vi "WSVCAP SHL Host TL Tester.vi"(0 "FPGA":T4) -> ()   [LabVIEW 2017]
uses:
  WSVCAP Shell Host Low Level/Host SRL/Type Defs/Cycle Pair Cluster.ctl
  Type Defs/WSVCAP SHL DUT Number Enum.ctl
  <vilib>/userdefined/High Color/nirio_resource_hc.ctl
  Type Defs/WSVCAP SHL FPGA Enum.ctl
  WSVCAP Shell Host Low Level/Host SRL/Type Defs/Cycle Instruction Cluster.ctl
  WSVCAP Shell Host Low Level/Host SRL/Type Defs/Cycle Scheme Enum.ctl
  Type Defs/Cap and DAC Table Manager Operation Enum.ctl
  Type Defs/WSVCAP SHL I2C DUT Mask Mode Enum.ctl
  WSVCAP Shell FPGA Low Level/FPGA-SRL/Debug Global.vi
  Type Defs/WSVCAP SHL Tester System Cluster.ctl
  WSVCAP Shell Host Low Level/Host SRL/Host SRL.lvlib
  WSVCAP Shell FPGA Low Level/FPGA-SRL/FPGA-SRL.lvlib
panel:
  in  "Cycle Scheme":T1
  in  "Cycle Pairs":T2[](array[typedef])=[{"G1 Ch (0-5)"=1, "G2 Ch (0-5)"=0, "En"=TRUE}, {"G1 Ch (0-5)"=3, "G2 Ch (0-5)"=2, "En"=TRUE}, {"G1 Ch (0-5)"=4, "G2 Ch (0-5)"=5, "En"=TRUE}] {"G2 Ch (0-5)" max=5 step=1 format="Ch %.0f"; "G1 Ch (0-5)" max=5 step=1 format="Ch %.0f"}
  in  "Vout 2 (V)":dbl=44.0 caption="Vout 2" format="%.3f V"
  in  "Device Ch (0-23)":u32
  in  "Data Out (14-bit)":u16 format="0x%04x"
  in  "Delay 2 (s)":dbl=5e-05 caption="Delay 2" format="%#_4ps"
  in  "Delay 1 (s)":dbl=5e-05 caption="Delay 1" format="%#_4ps"
  in  "Vout 1 (V)":dbl=44.0 caption="Vout 1" format="%.3f V"
  out "Cycle Count":u64=2 min=1 max=4 step=1
  out "Cycle Instructions":T3[](array[typedef]) {"Post CMD Delay (s)" format="%#_4ps"; "DAC Vout (V)" format="%.3f V"; "Dev Ch Idx (0-5)" max=5 step=1 format="Ch %d"}
  in  "Device Idx (0-5)":u32
  out "Dev Ch Idx (0-31)":u32 max=5 step=1 format="Dev Ch Idx: %d"
  out "Dev Idx (0-5)":u32 max=5 step=1 format="Dev Idx: %d"
  in  "DAC Out Vref (V)":dbl format="%.3f V"
  out "CMD [Hex]":u32 max=5 step=1 format="0x%05x"
  out "CMD [Bin]":u32 max=5 step=1 format="0b%019b"
  in  "Write DAC Voltage":bool
  in  "DUT Ch Idx (0-5)":u32 caption="DUT Ch Idx" max=5 step=1
  in  "DAC Vout (V)":dbl caption="Vout" format="%.3f V"
  in  "Cap DAC":u8=144 caption="B Data In" format="0x%02x"
  in  "Set Cap DAC":bool
  in  "Write Raw SRL":bool
  in  "Write Data DUT":string caption="Write Data Out"
  in  "Stop SRL Cycle":bool
  in  "Start SRL Cycle":bool
  in  "Monitor":bool
  out "AD7747 Values":string[][](table)
  in  "Mode":enum32{"All", "Single"}(radio)
  out "Activity Log":string
  out "Simulate FPGA":bool
  out "Online":bool
  out "FPGA Resource":T5
  out "Status":string
  out "Busy":bool
  in  "I2C Bytes to Read":u8=1 caption="Bytes" min=1 max=4 step=1
  in  "Exit":bool
  out "Read Data I2C":u8[](array[numeric]) caption="Data In" format="0x%02x"
  in  "Read Reg I2C":u8 caption="Register" format="0x%02x"
  in  "Read I2C":bool
  in  "DUT":T6
  in  "Write Data I2C":u8 caption="Data Out" format="0x%02x"
  in  "Write Reg I2C":u8=144 caption="Register" format="0x%02x"
  in  "I2C Init":bool
  in  "Init Data":u8[](array[numeric])=[164, 160, 14, 33] caption="Data Out" format="0x%02x"
  in  "Init Reg":u8[](array[numeric])=[191, 7, 9, 10] caption="Register" format="0x%02x"
  in  "Write I2C":bool
  in  "I2C Slave Address":u8=144 caption="Slave Address" format="0x%02x"
  in  "SRL Clock Rate (Hz)":dbl=1000000.0 caption="Clock Rate" format="%.1p Hz"
  in  "I2C Clock Rate (Hz)":dbl=100000.0 caption="Clock Rate" format="%.0p Hz"
  in  "Error":errorcluster
  # "WS1021 MEMS Only Tester"
  # "AD7747 (I2C)"
  # "C"
  # "DAC Control (SRL)"
  # "Vout Cycling (SRL)"
  # "Group 1"
  # "Group 2"
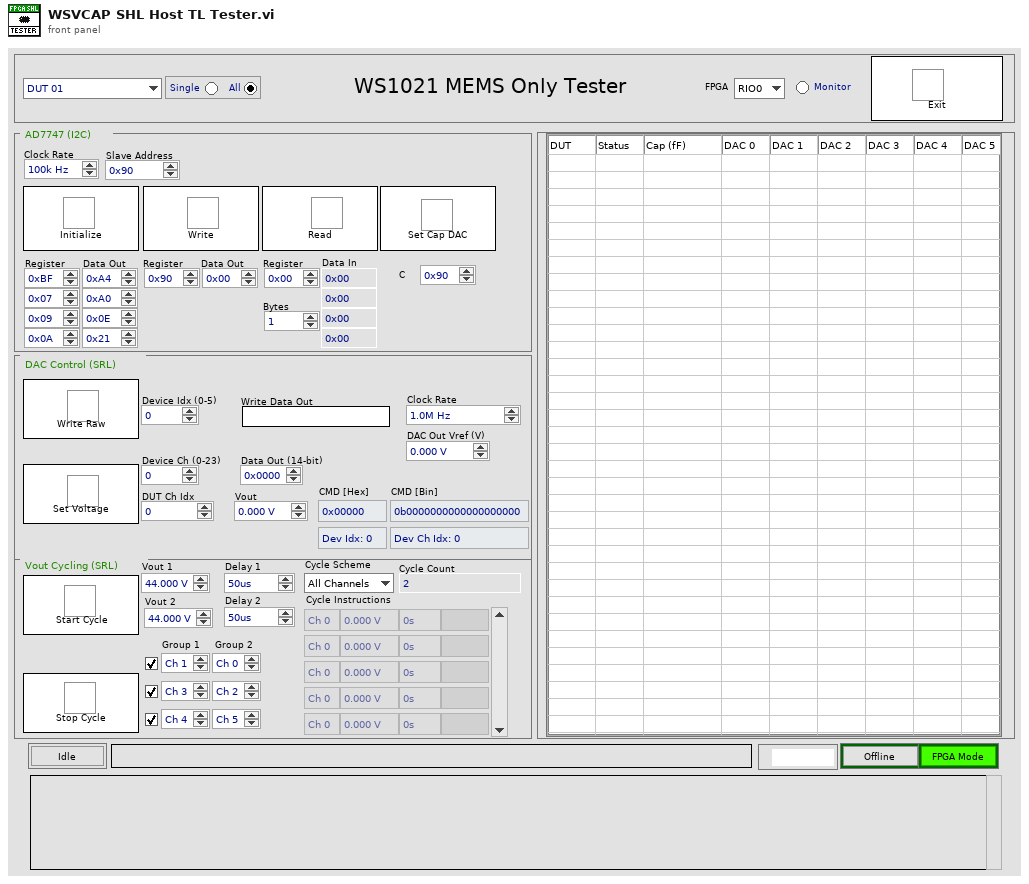
[diagram p1: front panel]
types:
  T1 = typedef "Cycle Scheme Enum.ctl" = enum16{"All Channels", "By Group"}
  T2 = typedef "Host SRL.lvlib/Cycle Pair Cluster.ctl" = cluster{"G1 Ch (0-5)":u32, "G2 Ch (0-5)":u32, "En":bool}
  T3 = typedef "Host SRL.lvlib/Cycle Instruction Cluster.ctl" = cluster{"Dev Ch Idx (0-5)":u32, "DAC Vout (V)":dbl, "Post CMD Delay (s)":dbl, "Raw CMD":string}
  T4 = typedef "WSVCAP SHL FPGA Enum.ctl" = enum16{"RIO0", "RIO1"}
  T5 = typedef "nirio_resource_hc.ctl" = tag
  T6 = typedef "WSVCAP SHL DUT Number Enum.ctl" = enum16{"DUT 01", "DUT 02", "DUT 03", "DUT 04", "DUT 05", "DUT 06", "DUT 07", "DUT 08", "DUT 09", "DUT 10", "DUT 11", "DUT 12", "DUT 13", "DUT 14", "DUT 15", "DUT 16", "DUT 17", "DUT 18", "DUT 19", "DUT 20", "DUT 21", "DUT 22", "DUT 23", "DUT 24"}
  T7 = typedef "Cap and DAC Table Manager Operation Enum.ctl" = enum16{"Initialize", "Add Single DAC", "Add All DAC", "Add All DUT Single DAC", "Add All Cap", "Get Status"}
  T8 = typedef "WSVCAP SHL Core System Cluster.ctl" = cluster{"Settings":T9, "FPGA Resource":tag, "Online":bool, "I2C Wait Ticks":u32, "SRL Wait Ticks":u32, "FPGA VI Reference (FPGA Mode)":T10, "FPGA VI Reference (Sim Mode)":refnum<vi>}
  T9 = typedef "WSVCAP SHL I2C Settings Cluster.ctl" = cluster{"I2C Slave Address":u8, "I2C Clock Rate (Hz)":dbl, "SRL Clock Rate (Hz)":dbl, "Simulate FPGA":bool, "C1 Cap DAC Default":u8, "C2 Cap DAC Default":u8, "C3 Cap DAC Default":u8, "C4 Cap DAC Default":u8, "DAC Out Vref (V)":dbl}
  T10 = typedef "WSVCAP SHL FPGA Ref.ctl" = refnum<k20>
  T11 = enum8{"Enabled", "Disabled", "Disabled and Grayed Out"}
  T12 = typedef "WSVCAP SHL I2C DUT Mask Mode Enum.ctl" = enum16{"Custom", "All"}
  T13 = typedef "WSVCAP SHL Tester System Cluster.ctl" = cluster{"I2C Monitor":bool, "SRL Cyle":bool, "DAC Vout (V)":dbl, "DUT Ch Idx (0-5)":u32, "Cycle Instructions":T3[], "Vout 1 (V)":dbl, "Delay 1 (s)":dbl, "Number of pairs":i32, "Delay 2 (s)":dbl, "Data Out (14-bit)":u16, "DUT":T6, "Vout 2 (V)":dbl, "Cycle Scheme":T1}
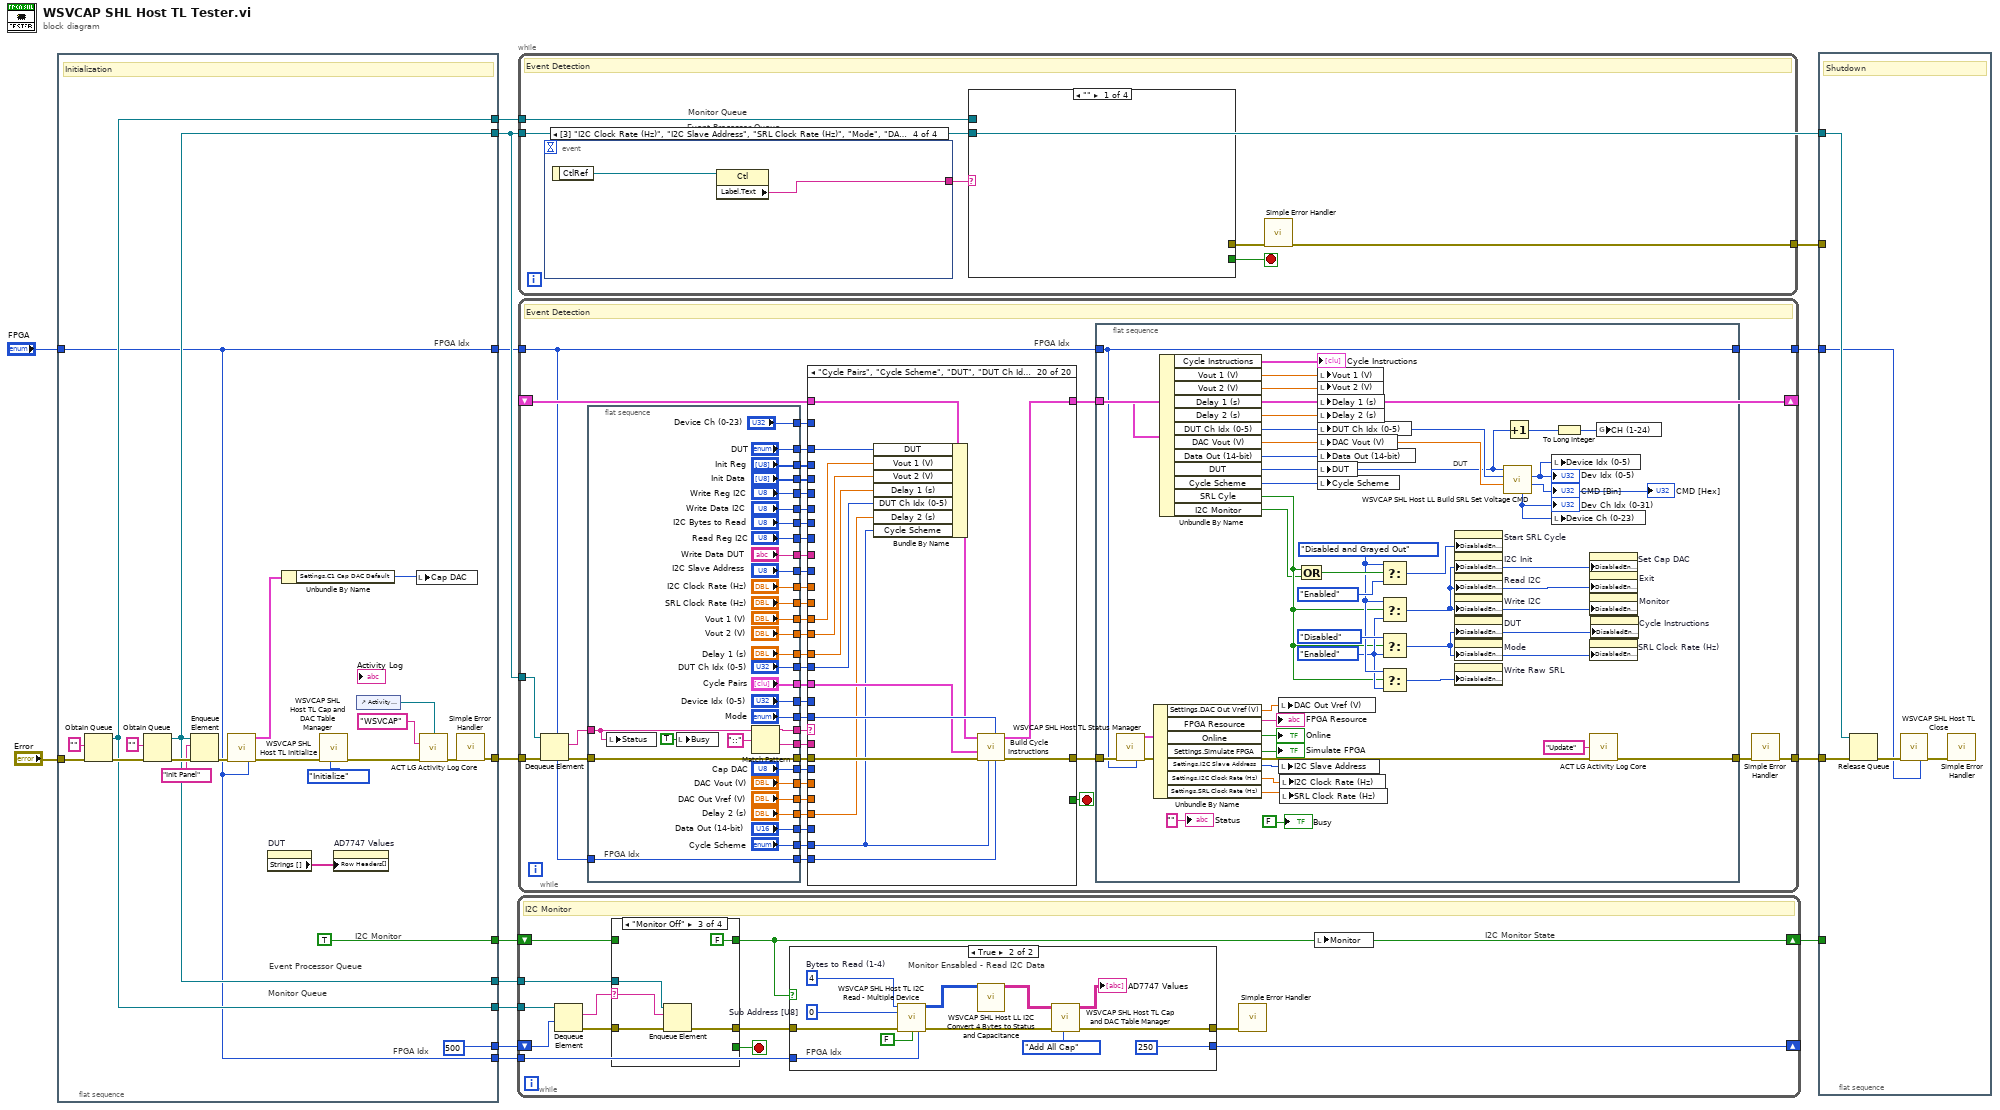
[diagram p0: block diagram]
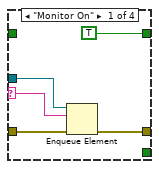
[diagram p2: hidden frame]
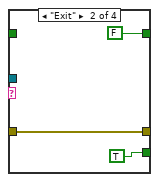
[diagram p3: hidden frame]
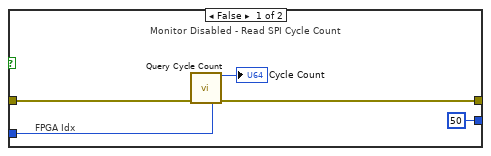
[diagram p5: hidden frame]
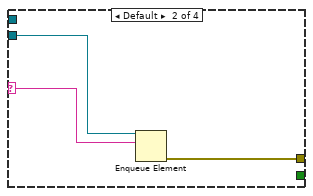
[diagram p6: hidden frame]
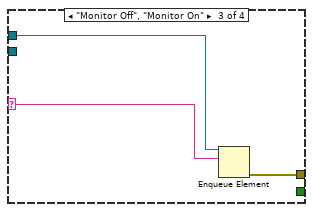
[diagram p7: hidden frame]
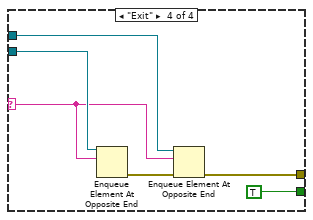
[diagram p8: hidden frame]
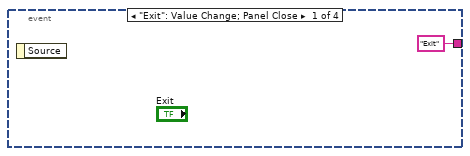
[diagram p9: hidden frame]
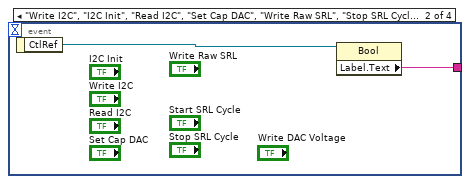
[diagram p10: hidden frame]
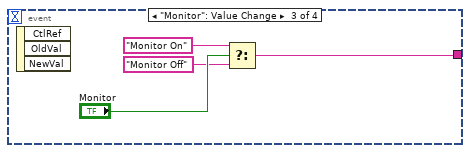
[diagram p11: hidden frame]
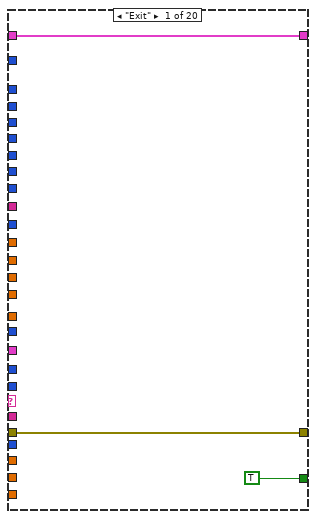
[diagram p12: hidden frame]
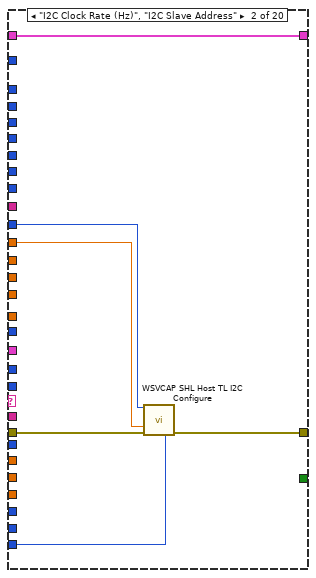
[diagram p13: hidden frame]
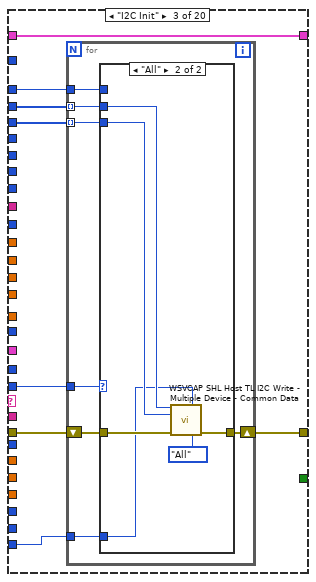
[diagram p14: hidden frame]
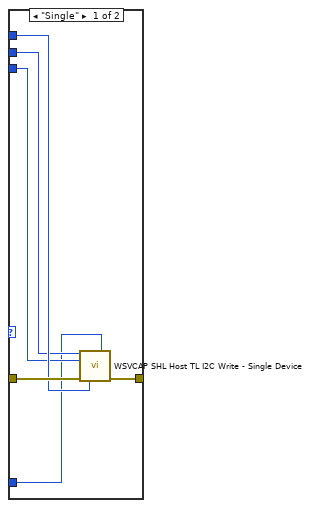
[diagram p15: hidden frame]
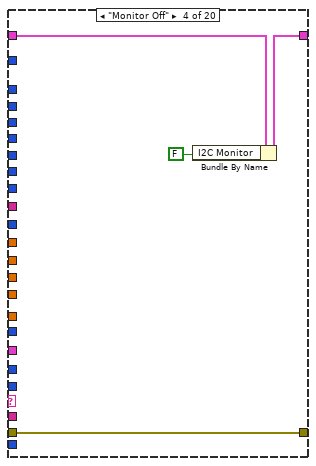
[diagram p16: hidden frame]
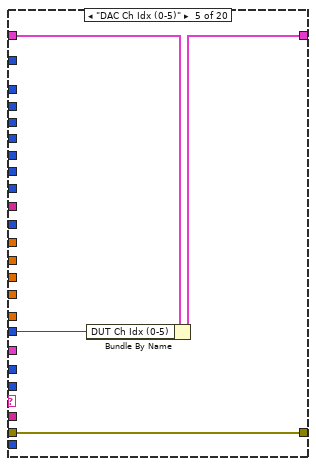
[diagram p17: hidden frame]
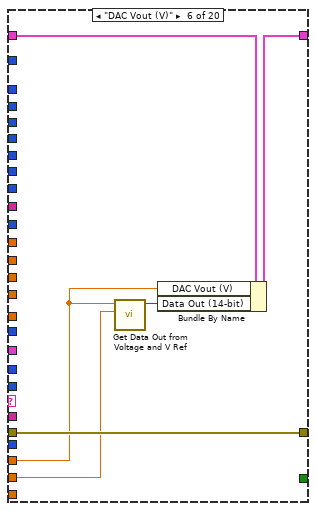
[diagram p18: hidden frame]
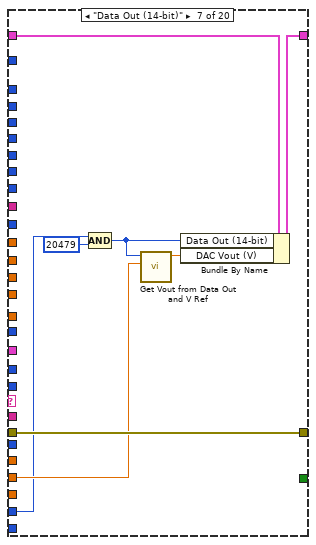
[diagram p19: hidden frame]
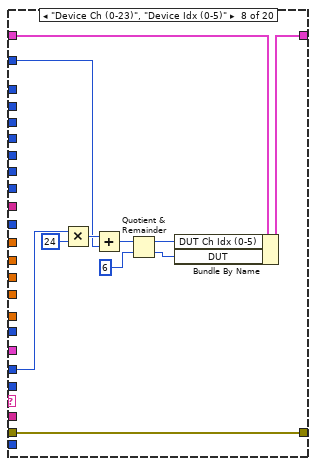
[diagram p20: hidden frame]
diagram:
  n1 = flat-sequence "Initialize" {
    tunnel: "Error" -> [w28]
    tunnel: [w26] -> w14
    tunnel: [TRUE ("Monitor")] -> w7
    tunnel: [w33] -> w11
    tunnel: [w25] -> w10
    tunnel: [w26] -> w9
    tunnel: [w25] -> w8
    tunnel: [500 ("Wait Time (500ms)")] -> w6
    tunnel: "FPGA" -> [w19]
    tunnel: [w19] -> w4
    tunnel: [w19] -> w2
    frame #0 {
      # "FPGA Idx"
      # "FPGA Idx"
      # "I2C Monitor"
      # "Monitor Queue"
      # "Event Processor Queue"
      # "Initialization"
      n2 = Obtain Queue(element data type="" ("name (unnamed)"), error in (no error)=w28) -> (queue out=w25:refnum<queue>, error out=w27:errorcluster)  [unwired: 3 in, 1 out]
      n3 = Obtain Queue(element data type="" ("name (unnamed)"), error in (no error)=w27) -> (queue out=w26:refnum<queue>, error out=w36:errorcluster)  [unwired: 3 in, 1 out]
      n4 = Enqueue Element(queue=w26, element="Init Panel" ("name (unnamed)"), error in (no error)=w36) -> (error out=w23:errorcluster)  [unwired: 1 in, 2 out]
      n5 = call "WSVCAP SHL Host TL Initialize.vi"("error in"=w23, "FPGA"=w19) -> ("System"=w22:T8, "error out"=w17:errorcluster)  [unwired: 12 in]
      n6 = property on="DUT" class="Enum (strict)"() -> ("Strings []"=w24:string[])  [unwired: 2 in, 2 out]
      n7 = Unbundle By Name(w22) -> ("Settings.C1 Cap DAC Default"=w21:u8)
      n8 = call "WSVCAP SHL Host TL Cap and DAC Table Manager.vi"("Operation"=Cap_and_DAC_Table_Manager_Operation_Enum."Initialize", "Error In"=w17) -> ("Error Out"=w16:errorcluster)  [unwired: 8 in, 1 out]
      n9 = property on="AD7747 Values" class="Tbl (strict)"("Row Headers[]"=w24) -> ()  [unwired: 2 in, 2 out]
      n10 = control-ref of="Activity Log"() -> (w32:refnum<vi>)
      n11 = local write "Cap DAC"(w21) -> ()
      n12 = call "ACT LG Activity Log Core.vi"("Display Ref"=w32, "Source"="WSVCAP", "Error In (no error)"=w16) -> ("Error Out"=w34:errorcluster)  [unwired: 11 in, 1 out]
      n13 = call <vilib>:"Simple Error Handler.vi"("error in (no error)"=w34) -> ("error out"=w33:errorcluster)  [unwired: 4 in, 4 out]
    }
  }
  n14 = while "Monitor" {
    shift-right: [w41] -> w1
    shift-left: w7 -> [w47]
    tunnel: w10 -> [w45]
    tunnel: w9 -> [w44]
    shift-right: [w40] -> _
    shift-left: w6 -> [w39]
    tunnel: w2 -> [w38]
    stop <- w42 stop-if-true
    # "I2C Monitor State"
    # "I2C Monitor"
    n15 = Dequeue Element(queue=w45, timeout in ms (-1)=w39) -> (element=w48:string, error out=w46:errorcluster)  [unwired: 1 in, 2 out]
    n16 = case shown="\"Monitor Off\"" w48 {
      selector: w48 -> [w51 _ w59 _]
      tunnel: [TRUE FALSE FALSE w64] -> w41
      tunnel: w47 -> [_ _ _ w64]
      tunnel: w46 -> [w53 w56 w61 w63]
      tunnel: [w52 w56 w60 w63] -> w43
      tunnel: w44 -> [w50 _ w58 _]
      tunnel: [_ TRUE _ _] -> w42
      frame "Monitor On" {
        n17 = Enqueue Element(queue=w50, element=w51, error in (no error)=w53) -> (error out=w52:errorcluster)  [unwired: 1 in, 2 out]
      }
      frame "Exit" {
      }
      frame "Monitor Off" {
        n18 = Enqueue Element(queue=w58, element=w59, error in (no error)=w61) -> (error out=w60:errorcluster)  [unwired: 1 in, 2 out]
      }
      frame Default {
      }
    }
    n19 = case shown="True" w41 {
      tunnel: [w67 w71] -> w49
      tunnel: w43 -> [w68 w78]
      tunnel: [50 ("Wait Time (500ms)") 250 ("Wait Time (500ms)")] -> w40
      tunnel: w38 -> [w65 w75]
      frame False {
        # "FPGA Idx"
        # "Monitor Disabled - Read SPI Cycle Count"
        n20 = call "Query Cycle Count.vi"("error in"=w68, "FPGA"=w65) -> ("Cycle Count"=→"Cycle Count":u64, "error out"=w67:errorcluster)  [unwired: 12 in]
      }
      frame True {
        w80 = u8 4  # Bytes to Read (1-4)
        w81 = u8 0  # Sub Address [U8]
        # "FPGA Idx"
        # "Monitor Ensabled - Read I2C Data"
        n21 = call "WSVCAP SHL Host TL I2C Read - Multiple Device.vi"("Bytes to Read (1-4)"=w80, "Sub Address [U8]"=w81, "error in"=w78, "Log (T)"=FALSE, "FPGA"=w75) -> ("C:1-24 Read Data [U8]"=w79:u8[][], "error out"=w72:errorcluster)  [unwired: 9 in]
        n22 = call "WSVCAP SHL Host LL I2C Convert 4 Bytes to Status and Capacitance.vi"("C:1-24 Read Data [U8]"=w79) -> ("AD7747 Values"=w74:string[][])  [unwired: 14 in]
        n23 = call "WSVCAP SHL Host TL Cap and DAC Table Manager.vi"("Operation"=Cap_and_DAC_Table_Manager_Operation_Enum."Add All Cap", "Error In"=w72, "Data In"=w74) -> ("Error Out"=w71:errorcluster, "Table Out"=→"AD7747 Values":string[][])  [unwired: 7 in]
      }
    }
    n24 = call <vilib>:"Simple Error Handler.vi"("error in (no error)"=w49) -> ()  [unwired: 4 in, 5 out]
    n25 = local write "Monitor"(w41) -> ()
  }
  n26 = while "User Interface Event Detector" {
    tunnel: w14 -> [w86]
    tunnel: [w83] -> w12
    tunnel: w8 -> [w82]
    stop <- w84 stop-if-true
    # "Monitor Queue"
    # "Event Processor Queue"
    # "Event Detection"
    n27 = event shown="[3] \"I2C Clock Rate (Hz)\", \"I2C Slave Address\", \"SRL Clock Rate (Hz)\", \"Mode\", \"DAC Out Vref (V)\", \"DUT Ch Idx (0-5)\", \"DAC Vout (V)\", \"DUT\", \"Vout 1 (V)\", \"Delay 1 (s)\", \"Cycle Pairs\", \"Data Out (14-bit)\", \"Device Ch (0-23)\", \"Delay 2 (s)\", \"Vout 2 (V)\", \"Cycle Scheme\": Value Change" {
      selector: _ -> [_ _ _ _]
      dyn-events: _ -> [_ _ _ _]
      timeout: _ -> [_ _ _ _]
      tunnel: ["Exit" ("Label.Text") w102 w103 w107] -> w87
      event "Exit": Value Change; Panel Close {
        n28 = event-data() -> ()  [unwired: 1 in, 1 out]
      }
      event "Write I2C", "I2C Init", "Read I2C", "Set Cap DAC", "Write Raw SRL", "Stop SRL Cycle", "Start SRL Cycle", "Write DAC Voltage": Value Change {
        n29 = event-data() -> ("CtlRef"=w101:refnum<vi>)  [unwired: 1 in]
        n30 = property class="Bool"(reference=w101) -> ("Label.Text"=w102:string)  [unwired: 1 in, 2 out]
      }
      event "Monitor": Value Change {
        n31 = event-data() -> ()  [unwired: 1 in, 3 out]
        n32 = Select(t="Monitor On" ("Label.Text"), s="Monitor", f="Monitor Off" ("Label.Text")) -> (s? t:f=w103:string)
      }
      event "I2C Clock Rate (Hz)", "I2C Slave Address", "SRL Clock Rate (Hz)", "Mode", "DAC Out Vref (V)", "DUT Ch Idx (0-5)", "DAC Vout (V)", "Vout 1 (V)", "Delay 1 (s)", "Cycle Pairs", "Data Out (14-bit)", "Device Ch (0-23)", "Delay 2 (s)", "Vout 2 (V)": Value Change {
        n33 = event-data() -> ("CtlRef"=w108:refnum<vi>)  [unwired: 1 in]
        n34 = property class="Ctl"(reference=w108) -> ("Label.Text"=w107:string)  [unwired: 1 in, 2 out]
      }
    }
    n35 = case shown="\"\"" w87 {
      selector: w87 -> [_ w90 w93 w94]
      tunnel: w86 -> [_ w89 _ w99]
      tunnel: [_ w88 w92 w96] -> w85
      tunnel: [_ _ _ TRUE] -> w84
      tunnel: w82 -> [_ _ w91 w95]
      frame "" {
      }
      frame Default {
        n36 = Enqueue Element(queue=w89, element=w90) -> (error out=w88:errorcluster)  [unwired: 2 in, 2 out]
      }
      frame "Monitor Off", "Monitor On" {
        n37 = Enqueue Element(queue=w91, element=w93) -> (error out=w92:errorcluster)  [unwired: 2 in, 2 out]
      }
      frame "Exit" {
        n38 = Enqueue Element At Opposite End(queue=w99, element=w94) -> (error out=w97:errorcluster)  [unwired: 2 in, 2 out]
        n39 = Enqueue Element At Opposite End(queue=w95, element=w94, error in (no error)=w97) -> (error out=w96:errorcluster)  [unwired: 1 in, 2 out]
      }
    }
    n40 = call <vilib>:"Simple Error Handler.vi"("error in (no error)"=w85) -> ("error out"=w83:errorcluster)  [unwired: 4 in, 4 out]
  }
  n41 = while "Event Processer" {
    tunnel: w14 -> [w149]
    tunnel: [w147] -> w13
    tunnel: w11 -> [w130]
    shift-right: [w128] -> _
    shift-left: _ -> [w129]
    tunnel: w4 -> [w123]
    tunnel: [w109] -> w3
    stop <- w148 stop-if-true
    # "FPGA Idx"
    # "Event Detection"
    n42 = Dequeue Element(queue=w149, error in (no error)=w130) -> (element=w145:string, error out=w143:errorcluster)  [unwired: 1 in, 2 out]
    n43 = flat-sequence {
      tunnel: ["I2C Clock Rate (Hz)"] -> w146
      tunnel: [w208] -> w144
      tunnel: w145 -> [w209]
      tunnel: [w222] -> w142
      tunnel: w143 -> [w222]
      tunnel: ["I2C Bytes to Read"] -> w141
      tunnel: ["I2C Slave Address"] -> w140
      tunnel: ["SRL Clock Rate (Hz)"] -> w139
      tunnel: ["DUT"] -> w122
      tunnel: ["Init Data"] -> w136
      tunnel: ["Init Reg"] -> w135
      tunnel: ["Write Reg I2C"] -> w134
      tunnel: ["Write Data I2C"] -> w133
      tunnel: ["Read Reg I2C"] -> w132
      tunnel: ["Write Data DUT"] -> w131
      tunnel: ["Mode"] -> w127
      tunnel: [w206] -> w126
      tunnel: ["Cap DAC"] -> w125
      tunnel: [w204] -> w124
      tunnel: w123 -> [w204]
      tunnel: ["DUT Ch Idx (0-5)"] -> w120
      tunnel: ["DAC Vout (V)"] -> w121
      tunnel: ["DAC Out Vref (V)"] -> w119
      tunnel: ["Device Idx (0-5)"] -> w118
      tunnel: ["Vout 1 (V)"] -> w117
      tunnel: ["Delay 1 (s)"] -> w116
      tunnel: ["Cycle Pairs"] -> w115
      tunnel: ["Delay 2 (s)"] -> w114
      tunnel: ["Data Out (14-bit)"] -> w113
      tunnel: ["Device Ch (0-23)"] -> w112
      tunnel: ["Vout 2 (V)"] -> w111
      tunnel: ["Cycle Scheme"] -> w110
      frame #0 {
        # "FPGA Idx"
        n44 = local write "Status"(w209) -> ()
        n45 = local write "Busy"(TRUE ("Busy")) -> ()
        n46 = Match Pattern(string=w209, regular expression="::") -> (before substring=w208:string, after substring=w206:string)  [unwired: 1 in, 2 out]
      }
    }
    n47 = case shown="\"Cycle Pairs\", \"Cycle Scheme\", \"DUT\", \"DUT Ch Idx (0-5)\", \"Delay 1 (s)\", \"Delay 2 (s)\", \"Mode\", \"Number of Pairs\", \"Vout 1 (V)\", \"Vout 2 (V)\"" w144 {
      tunnel: w142 -> [w225 w232 w240 w263 w267 w273 w281 w292 w297 w305 w311 w317 w327 w348 w371 w386 w394 w408 w415 w429]
      tunnel: [w225 w229 w239 w263 w267 w273 w281 w292 w297 w300 w309 w316 w326 w342 w370 w385 w393 w408 w415 w428] -> w138
      tunnel: [TRUE _ _ _ _ _ _ _ _ _ _ _ _ _ _ _ _ _ _ _] -> w148
      tunnel: w146 -> [_ w231 _ _ _ _ _ _ _ _ _ _ _ _ _ _ _ _ _ _]
      tunnel: w141 -> [_ _ _ _ _ _ _ _ _ w302 _ _ _ _ _ _ _ _ _ _]
      tunnel: w140 -> [_ w230 _ _ _ _ _ _ _ _ _ _ _ _ _ _ _ _ _ _]
      tunnel: w139 -> [_ _ _ _ _ _ _ _ _ _ w310 _ _ _ _ _ _ _ _ _]
      tunnel: w122 -> [_ _ w237 _ _ _ _ _ _ w304 _ _ w321 w344 w365 _ w391 _ _ w423]
      tunnel: w136 -> [_ _ w235 _ _ _ _ _ _ _ _ _ _ _ _ _ _ _ _ _]
      tunnel: w135 -> [_ _ w236 _ _ _ _ _ _ _ _ _ _ _ _ _ _ _ _ _]
      tunnel: w134 -> [_ _ _ _ _ _ _ _ _ _ _ _ _ _ _ _ w390 _ _ _]
      tunnel: w133 -> [_ _ _ _ _ _ _ _ _ _ _ _ _ _ _ _ w389 _ _ _]
      tunnel: w132 -> [_ _ _ _ _ _ _ _ _ w303 _ _ _ _ _ _ _ _ _ _]
      tunnel: w131 -> [_ _ _ _ _ _ _ _ _ _ _ _ w324 _ _ _ _ _ _ _]
      tunnel: w127 -> [_ _ w238 _ _ _ _ _ _ _ _ _ w325 w337 w369 _ w392 _ _ w430]
      tunnel: [w224 w228 w234 w261 w265 w271 w279 w290 w295 w299 w308 w319 w323 w349 w368 w382 w388 w407 w412 w419] -> w128
      tunnel: w129 -> [w224 w228 w234 w262 w266 w272 w280 w291 w296 w299 w308 w319 w323 w349 w364 w383 w388 w407 w410 w432]
      tunnel: w126 -> [_ _ _ _ _ _ _ _ _ _ _ _ _ _ _ _ _ _ _ _]
      tunnel: w125 -> [_ _ _ _ _ _ _ _ _ _ _ w315 _ _ _ _ _ _ _ _]
      tunnel: w124 -> [_ w227 w233 _ _ _ _ _ _ w298 w307 w314 w322 w343 w366 w381 w387 _ _ w431]
      tunnel: w120 -> [_ _ _ _ w264 _ _ _ _ _ _ _ _ w347 _ _ _ _ _ w427]
      tunnel: w121 -> [_ _ _ _ _ w270 _ _ _ _ _ _ _ w346 _ _ _ _ _ _]
      tunnel: w119 -> [_ _ _ _ _ w269 w278 _ _ _ w306 _ _ w345 _ _ _ _ _ _]
      tunnel: w118 -> [_ _ _ _ _ _ _ w289 _ _ _ _ w320 _ _ _ _ _ _ _]
      tunnel: w117 -> [_ _ _ _ _ _ _ _ _ _ _ _ _ _ _ _ _ _ _ w426]
      tunnel: w116 -> [_ _ _ _ _ _ _ _ _ _ _ _ _ _ _ _ _ _ _ w425]
      tunnel: w115 -> [_ _ _ _ _ _ _ _ _ _ _ _ _ _ _ _ _ _ _ w424]
      tunnel: w114 -> [_ _ _ _ _ _ _ _ _ _ _ _ _ _ _ _ _ _ _ w422]
      tunnel: w113 -> [_ _ _ _ _ _ w276 _ _ _ _ _ _ _ _ _ _ _ _ _]
      tunnel: w112 -> [_ _ _ _ _ _ _ w286 _ _ _ _ _ _ _ _ _ _ _ _]
      tunnel: w111 -> [_ _ _ _ _ _ _ _ _ _ _ _ _ _ _ _ _ _ _ w421]
      tunnel: w110 -> [_ _ _ _ _ _ _ _ _ _ _ _ _ _ _ _ _ _ _ w418]
      frame "Exit" {
      }
      frame "I2C Clock Rate (Hz)", "I2C Slave Address" {
        n48 = call "WSVCAP SHL Host TL I2C Configure.vi"("I2C_Slave Address"=w230, "Clock Rate (Hz)"=w231, "error in"=w232, "FPGA"=w227) -> ("error out"=w229:errorcluster)  [unwired: 10 in, 1 out]
      }
      frame "I2C Init" {
        n49 = for {
          tunnel: w238 -> [w245]
          tunnel: w237 -> [w244]
          tunnel: w236 -> [w243] mode=indexing
          tunnel: w235 -> [w242] mode=indexing
          shift-right: [w246] -> w239
          shift-left: w240 -> [w247]
          tunnel: w233 -> [w241]
          n50 = case shown="\"All\"" w245 {
            tunnel: w247 -> [w253 w259]
            tunnel: [w252 w258] -> w246
            tunnel: w244 -> [w251 _]
            tunnel: w243 -> [w250 w257]
            tunnel: w242 -> [w249 w256]
            tunnel: w241 -> [w248 w255]
            frame "Single" {
              n51 = call "WSVCAP SHL Host TL I2C Write - Single Device.vi"("Sub Address [U8]"=w250, "FPGA"=w248, "Data Out [U8]"=w249, "error in"=w253, "DUT"=w251) -> ("error out"=w252:errorcluster)  [unwired: 10 in]
            }
            frame "All" {
              n52 = call "WSVCAP SHL Host TL I2C Write - Multiple Device - Common Data.vi"("Sub Address"=w257, "FPGA"=w255, "Data Out [U8]"=w256, "error in"=w259, "DUT Mask Mode (All)"=WSVCAP_SHL_I2C_DUT_Mask_Mode_Enum."All") -> ("error out"=w258:errorcluster)  [unwired: 10 in]
            }
          }
        }
      }
      frame "Monitor Off" {
        n53 = Bundle By Name(cluster=w262, "I2C Monitor"=FALSE) -> (w261:T13)
      }
      frame "DAC Ch Idx (0-5)" {
        n54 = Bundle By Name(cluster=w266, "DUT Ch Idx (0-5)"=w264) -> (w265:T13)
      }
      frame "DAC Vout (V)" {
        n55 = call "Get Data Out from Voltage and V Ref.vi"("Vref (V)"=w269, "Voltage (V)"=w270) -> ("Data Out (14-bit)"=w268:u16)  [unwired: 9 in]
        n56 = Bundle By Name(cluster=w272, "DAC Vout (V)"=w270, "Data Out (14-bit)"=w268) -> (w271:T13)
      }
      frame "Data Out (14-bit)" {
        n57 = Compound Arithmetic op=AND(w276, u16 20479 ("value")) -> (w274:u16)
        n58 = call "Get Vout from Data Out and V Ref.vi"("Vref"=w278, "Data out (14-bit)"=w274) -> ("Vout (V)"=w277:dbl)  [unwired: 9 in]
        n59 = Bundle By Name(cluster=w280, "Data Out (14-bit)"=w274, "DAC Vout (V)"=w277) -> (w279:T13)
      }
      frame "Device Ch (0-23)", "Device Idx (0-5)" {
        n60 = Multiply(x=w289, y=u32 24) -> (x*y=w287:u32)
        n61 = Add(x=w287, y=w286) -> (x+y=w285:u32)
        n62 = Quotient & Remainder(x=w285, y=u32 6) -> (x-y*floor(x/y)=w283:u32, floor(x/y)=w282:u32)
        n63 = Bundle By Name(cluster=w291, "DUT Ch Idx (0-5)"=w283, "DUT"=w282) -> (w290:T13)
      }
      frame "Monitor On" {
        n64 = Bundle By Name(cluster=w296, "I2C Monitor"=TRUE, "SRL Cyle"=FALSE ("I2C Monitor")) -> (w295:T13)
      }
      frame "Read I2C" {
        n65 = call "WSVCAP SHL Host TL I2C Read - Single Device.vi"("Bytes to Read (1-4)"=w302, "FPGA"=w298, "Sub Address [U8]"=w303, "error in"=w305, "DUT"=w304) -> ("Device Data"=→"Read Data I2C":u8[], "error out"=w300:errorcluster)  [unwired: 9 in]
      }
      frame "DAC Out Vref (V)", "SRL Clock Rate (Hz)" {
        n66 = call "Configure.vi"("Vref (V)"=w306, "Clock Rate (Hz)"=w310, "error in"=w311, "FPGA"=w307) -> ("error out"=w309:errorcluster)  [unwired: 10 in, 1 out]
      }
      frame "Set Cap DAC" {
        n67 = Initialize Array(w315, 64 ("dimension size")) -> (w318:u8[])
        n68 = call "WSVCAP SHL Host TL I2C Write - Multiple Device - Unique Data.vi"("C1 Data"=w318, "Sub Address"=u8 11, "FPGA"=w314, "error in"=w317) -> ("error out"=w316:errorcluster)  [unwired: 11 in]
      }
      frame "Write Raw SRL" {
        n69 = case shown="\"Single\"" w325 {
          tunnel: w327 -> [w332 w336]
          tunnel: [w330 w335] -> w326
          tunnel: w321 -> [_ _]
          tunnel: w324 -> [w331 w334]
          tunnel: w322 -> [w329 w333]
          tunnel: w320 -> [w328 _]
          frame "Single" {
            n70 = call "Write Raw CMD - Single Device.vi"("Data Out"=w331, "error in"=w332, "Device Idx (0-5)"=w328, "FPGA"=w329) -> ("error out"=w330:errorcluster)  [unwired: 11 in]
          }
          frame "All" {
            n71 = call "Write Raw CMD - Multiple Devices - Common Data.vi"("Raw CMD"=w334, "error in"=w336, "FPGA"=w333) -> ("error out"=w335:errorcluster)  [unwired: 12 in]
          }
        }
      }
      frame "Write DAC Voltage" {
        n72 = case shown="\"All\"" w337 {
          tunnel: w348 -> [w356 w362]
          tunnel: w347 -> [w355 w361]
          tunnel: w346 -> [w354 w360]
          tunnel: w345 -> [w353 w359]
          tunnel: w344 -> [w352 _]
          tunnel: w343 -> [w351 w358]
          tunnel: [w350 w357] -> w341
          frame "Single" {
            n73 = call "Write DAC Voltage - Single DUT.vi"("Channel (0-5)"=w355, "Voltage"=w354, "Vref (-1: Unchanged)"=w353, "error in"=w356, "DUT"=w352, "FPGA"=w351) -> ("error out"=w350:errorcluster)  [unwired: 8 in, 1 out]
          }
          frame "All" {
            n74 = call "Write DAC Voltage - All DUTs - Single Channel.vi"("Channel (0-5)"=w361, "Voltage"=w360, "Vref (-1: Unchanged)"=w359, "error in"=w362, "FPGA"=w358) -> ("error out"=w357:errorcluster)  [unwired: 9 in, 1 out]
          }
        }
        n75 = call "WSVCAP SHL Host TL Cap and DAC Table Manager.vi"("Operation"=Cap_and_DAC_Table_Manager_Operation_Enum."Get Status", "Error In"=w341) -> ("Error Out"=w340:errorcluster, "Table Out"=w339:string[][])  [unwired: 8 in]
        n76 = property on="AD7747 Values" class="Tbl (strict)"(error in=w340, "Value"=w339) -> (error out=w342:errorcluster)  [unwired: 1 in, 1 out]
      }
      frame "Start SRL Cycle" {
        n77 = Unbundle By Name(w364) -> ("Cycle Instructions"=w363:T3[])
        n78 = case shown="\"Single\"" w369 {
          tunnel: w371 -> [w376 w380]
          tunnel: [w375 w379] -> w370
          tunnel: w363 -> [w374 w378]
          tunnel: w366 -> [w373 w377]
          tunnel: w365 -> [w372 _]
          frame "Single" {
            n79 = call "Write Cycle - Single DUT.vi"("Cycle Instructions"=w374, "error in"=w376, "DUT"=w372, "FPGA"=w373) -> ("error out"=w375:errorcluster)  [unwired: 11 in]
          }
          frame "All" {
            n80 = call "Write Cycle - Multiple DUTs - Common Data.vi"("Cycle Instructions"=w378, "error in"=w380, "FPGA"=w377) -> ("error out"=w379:errorcluster)  [unwired: 12 in]
          }
        }
        n81 = Bundle By Name(cluster=w364, "SRL Cyle"=TRUE ("SPI Cyle")) -> (w368:T13)
      }
      frame "Stop SRL Cycle" {
        n82 = call "Stop Write Cycle.vi"("error in"=w386, "FPGA"=w381) -> ("error out"=w385:errorcluster)  [unwired: 13 in]
        n83 = Bundle By Name(cluster=w383, "SRL Cyle"=FALSE ("SPI Cyle")) -> (w382:T13)
      }
      frame "Write I2C" {
        n84 = case shown="\"Single\"" w392 {
          tunnel: w394 -> [w400 w406]
          tunnel: [w399 w405] -> w393
          tunnel: w391 -> [w398 _]
          tunnel: w390 -> [w397 w404]
          tunnel: w389 -> [w396 w403]
          tunnel: w387 -> [w395 w402]
          frame "Single" {
            n85 = call "WSVCAP SHL Host TL I2C Write - Single Device.vi"("Sub Address [U8]"=w397, "FPGA"=w395, "Data Out [U8]"=w396, "error in"=w400, "DUT"=w398) -> ("error out"=w399:errorcluster)  [unwired: 10 in]
          }
          frame "All" {
            n86 = call "WSVCAP SHL Host TL I2C Write - Multiple Device - Common Data.vi"("Sub Address"=w404, "FPGA"=w402, "Data Out [U8]"=w403, "error in"=w406, "DUT Mask Mode (All)"=WSVCAP_SHL_I2C_DUT_Mask_Mode_Enum."All") -> ("error out"=w405:errorcluster)  [unwired: 10 in]
          }
        }
      }
      frame Default {
      }
      frame "Init Panel" {
        n87 = case shown="True" FALSE {
          tunnel: [w416 T13 {"I2C Monitor"=TRUE, "SRL Cyle"=TRUE, "DAC Vout (V)"=0.0, "DUT Ch Idx (0-5)"=0, "Cycle Instructions"=[], "Vout 1 (V)"=0.0, "Delay 1 (s)"=0.0, "Number of pairs"=2, "Delay 2 (s)"=0.0, "Data Out (14-bit)"=0, "DUT"=enum."DUT 01", "Vout 2 (V)"=0.0, "Cycle Scheme"=enum."All Channels"} ("System")] -> w411
          tunnel: w410 -> [w416 _]
          frame False {
            # "For Type Only"
          }
          frame True {
          }
        }
        n88 = Bundle By Name(cluster=w411, "I2C Monitor"=TRUE, "SRL Cyle"=FALSE ("I2C Monitor")) -> (w412:T13)
      }
      frame "Cycle Pairs", "Cycle Scheme", "DUT", "DUT Ch Idx (0-5)", "Delay 1 (s)", "Delay 2 (s)", "Mode", "Number of Pairs", "Vout 1 (V)", "Vout 2 (V)" {
        n89 = Bundle By Name(cluster=w432, "DUT"=w423, "Vout 1 (V)"=w426, "Vout 2 (V)"=w421, "Delay 1 (s)"=w425, "DUT Ch Idx (0-5)"=w427, "Delay 2 (s)"=w422, "Cycle Scheme"=w418) -> (w420:T13)
        n90 = call "Build Cycle Instructions.vi"("FPGA"=w431, "DUT Mode"=w430, "Cycle Scheme"=w418, "error in"=w429, "Cycle Pairs"=w424, "System In"=w420) -> ("error out"=w428:errorcluster, "System Out"=w419:T13)  [unwired: 3 in, 1 out]
      }
    }
    n91 = flat-sequence {
      tunnel: [w179] -> w137
      tunnel: w138 -> [w189]
      tunnel: w128 -> [w178]
      tunnel: w123 -> [w151]
      tunnel: [w151] -> w109
      frame #0 {
        w173 = T11."Enabled" ("Disabled")
        w174 = T11."Disabled and Grayed Out" ("Disabled")
        # "DUT"
        n92 = call "WSVCAP SHL Host TL Status Manager.vi"("error in"=w189, "FPGA"=w151) -> ("System Out"=w188:T8, "error out"=w181:errorcluster)  [unwired: 12 in]
        n93 = Unbundle By Name(w188) -> ("Settings.DAC Out Vref (V)"=w168:dbl, "FPGA Resource"=→"FPGA Resource":tag, "Online"=→"Online":bool, "Settings.Simulate FPGA"=→"Simulate FPGA":bool, "Settings.I2C Slave Address"=w187:u8, "Settings.I2C Clock Rate (Hz)"=w186:dbl, "Settings.SRL Clock Rate (Hz)"=w185:dbl)
        n94 = Unbundle By Name(w178) -> ("Cycle Instructions"=→"Cycle Instructions":T3[], "Vout 1 (V)"=w159:dbl, "Vout 2 (V)"=w152:dbl, "Delay 1 (s)"=w158:dbl, "Delay 2 (s)"=w157:dbl, "DUT Ch Idx (0-5)"=w164:u32, "DAC Vout (V)"=w165:dbl, "Data Out (14-bit)"=w156:u16, "DUT"=w154:T6, "Cycle Scheme"=w150:T1, "SRL Cyle"=w162:bool, "I2C Monitor"=w161:bool)
        n95 = local write "DAC Out Vref (V)"(w168) -> ()
        n96 = local write "I2C Slave Address"(w187) -> ()
        n97 = local write "I2C Clock Rate (Hz)"(w186) -> ()
        n98 = local write "SRL Clock Rate (Hz)"(w185) -> ()
        n99 = Compound Arithmetic op=OR(w162, w161) -> (w175:bool)
        n100 = local write "Vout 1 (V)"(w159) -> ()
        n101 = local write "Vout 2 (V)"(w152) -> ()
        n102 = local write "Delay 1 (s)"(w158) -> ()
        n103 = local write "Delay 2 (s)"(w157) -> ()
        n104 = local write "DUT Ch Idx (0-5)"(w164) -> ()
        n105 = local write "DAC Vout (V)"(w165) -> ()
        n106 = local write "Data Out (14-bit)"(w156) -> ()
        n107 = local write "DUT"(w154) -> ()
        n108 = local write "Cycle Scheme"(w150) -> ()
        n109 = Select(t=w174, s=w175, f=T11."Enabled" ("Disabled")) -> (s? t:f=w172:T11)
        n110 = Select(t=w174, s=w162, f=w173) -> (s? t:f=w171:T11)
        n111 = Select(t=T11."Disabled" ("Disabled"), s=w162, f=w173) -> (s? t:f=w163:T11)
        n112 = Select(t=w174, s=w162, f=w173) -> (s? t:f=w170:T11)
        n113 = property on="Start SRL Cycle" class="Bool"("DisabledEnum"=w172) -> ()  [unwired: 2 in, 2 out]
        n114 = property on="I2C Init" class="Bool"("DisabledEnum"=w171) -> ()  [unwired: 2 in, 2 out]
        n115 = property on="Read I2C" class="Bool"("DisabledEnum"=w171) -> ()  [unwired: 2 in, 2 out]
        n116 = property on="Write I2C" class="Bool"("DisabledEnum"=w171) -> ()  [unwired: 2 in, 2 out]
        n117 = property on="DUT" class="Enum (strict)"("DisabledEnum"=w163) -> ()  [unwired: 2 in, 2 out]
        n118 = property on="Mode" class="RadioBtnsControl (strict)"("DisabledEnum"=w163) -> ()  [unwired: 2 in, 2 out]
        n119 = property on="Write Raw SRL" class="Bool"("DisabledEnum"=w170) -> ()  [unwired: 2 in, 2 out]
        n120 = call "WSVCAP SHL Host LL Build SRL Set Voltage CMD.vi"("Voltage (-1: Use Data Out)"=w165, "Channel (0-5)"=w164, "DUT"=w154) -> ("Raw CMD [Hex]"=→"CMD [Bin]" →"CMD [Hex]":u32, "Dev Idx (0-5)"=w153:u32, "Device Ch Idx (0-31)"=w155:u32)  [unwired: 4 in, 2 out]
        "Dev Idx (0-5)" <- w153
        "Dev Ch Idx (0-31)" <- w155
        n121 = Increment(x=w154) -> (x+1=w167:T6)
        n122 = local write "Device Idx (0-5)"(w153) -> ()
        n123 = local write "Device Ch (0-23)"(w155) -> ()
        n124 = To Long Integer(number=w167) -> (32bit integer=w166:i32)
        n125 = property on="Set Cap DAC" class="Bool"("DisabledEnum"=w171) -> ()  [unwired: 2 in, 2 out]
        n126 = property on="Exit" class="Bool"("DisabledEnum"=w171) -> ()  [unwired: 2 in, 2 out]
        n127 = property on="Monitor" class="Bool (strict)"("DisabledEnum"=w171) -> ()  [unwired: 2 in, 2 out]
        n128 = property on="SRL Clock Rate (Hz)" class="DigNum (strict)"("DisabledEnum"=w163) -> ()  [unwired: 2 in, 2 out]
        n129 = call "ACT LG Activity Log Core.vi"("Log Line"="Update", "Error In (no error)"=w181) -> ("Error Out"=w179:errorcluster)  [unwired: 12 in, 1 out]
        n130 = property on="Cycle Instructions" class="Arr (strict)"("DisabledEnum"=w163) -> ()  [unwired: 2 in, 2 out]
        n131 = global write "Debug Global.vi" "CH (1-24)"(w166) -> ()
        "Busy" <- FALSE ("Busy")
        "Status" <- "" ("Status")
      }
    }
    n132 = call <vilib>:"Simple Error Handler.vi"("error in (no error)"=w137) -> ("error out"=w147:errorcluster)  [unwired: 4 in, 4 out]
  }
  n133 = flat-sequence "Shutdown" {
    tunnel: w14 -> [w437]
    tunnel: w13 -> [w436]
    tunnel: w12 -> [_]
    tunnel: w3 -> [w433]
    tunnel: w1 -> [_]
    frame #0 {
      # "Shutdown"
      n134 = Release Queue(queue=w437, error in (no error)=w436) -> (error out=w435:errorcluster)  [unwired: 1 in, 2 out]
      n135 = call "WSVCAP SHL Host TL Close.vi"("error in"=w435, "FPGA"=w433) -> ("error out"=w434:errorcluster)  [unwired: 13 in]
      n136 = call <vilib>:"Simple Error Handler.vi"("error in (no error)"=w434) -> ()  [unwired: 4 in, 5 out]
    }
  }
